vi "MoveWithStick.vi"(8 "error in (no error)":errorcluster, 9 "DirectionY":i8, 10 "DirectionX":i8, 11 "PongPanel in":refnum<class "PongPanel.lvclass">) -> (0 "error out":errorcluster, 3 "PongPanel out":refnum<class "PongPanel.lvclass">)   [LabVIEW 2019, in "RT_Game.lvlib" / "PongPanel.lvclass"]
uses:
  PongPanel.lvclass
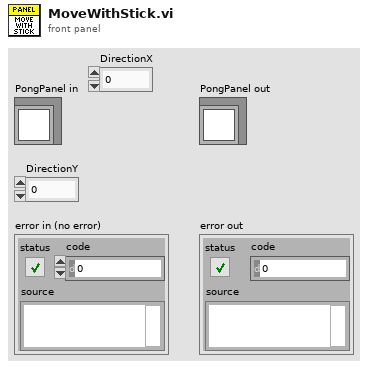
[diagram p1: front panel]
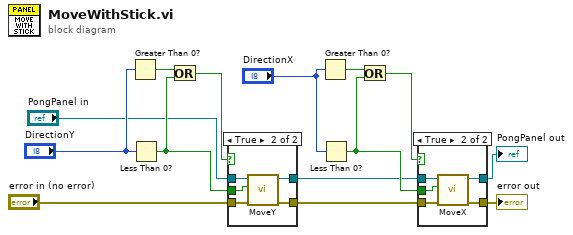
[diagram p0: block diagram]
diagram:
  n1 = Greater Than 0?(x="DirectionY") -> (x > 0?=w12:bool)
  n2 = Less Than 0?(x="DirectionY") -> (x < 0?=w14:bool)
  n3 = Or(x=w12, y=w14) -> (x .or. y?=w13:bool)
  n4 = case shown="True" w13 {
    tunnel: "error in (no error)" -> [w16 w21]
    tunnel: [w16 w20] -> w5
    tunnel: "PongPanel in" -> [w15 w19]
    tunnel: [w15 w18] -> w2
    tunnel: w14 -> [_ w17]
    frame False {
    }
    frame True {
      n5 = call "MoveY.vi"("error in (no error)"=w21, "Up?"=w17, "PongPanel in"=w19) -> ("error out"=w20:errorcluster, "PongPanel out"=w18:refnum<class "PongPanel.lvclass">)  [unwired: 7 in]
    }
  }
  n6 = Greater Than 0?(x="DirectionX") -> (x > 0?=w8:bool)
  n7 = Less Than 0?(x="DirectionX") -> (x < 0?=w6:bool)
  n8 = Or(x=w8, y=w6) -> (x .or. y?=w7:bool)
  n9 = case shown="True" w7 {
    tunnel: w5 -> [w23 w28]
    tunnel: [w23 w27] -> w4
    tunnel: w2 -> [w22 w26]
    tunnel: [w22 w25] -> w3
    tunnel: w6 -> [_ w24]
    frame False {
    }
    frame True {
      n10 = call "MoveX.vi"("error in (no error)"=w28, "Left?"=w24, "PongPanel in"=w26) -> ("error out"=w27:errorcluster, "PongPanel out"=w25:refnum<class "PongPanel.lvclass">)  [unwired: 7 in]
    }
  }
  "PongPanel out" <- w3
  "error out" <- w4
